vi "ClearLastError.vi"(8 "error in (no error)":errorcluster, 11 "session id in":i32) -> (0 "error out":errorcluster, 3 "session id out":i32)   [LabVIEW 2018, in "libonnx_wrapper.lvlib"]
doc: "/**\n * @brief Очистить сообщение об ошибке для сессии\n * \n * Сбрасывает сохраненное сообщение об ошибке. Полезно после обработки ошибки,\n * чтобы не получить старое сообщение при следующей проверке.\n * \n * @param sessionId [IN] ID сессии\n * \n * @return void\n */\nvoid ClearLastError(int sessionId);"
uses:
  libonnx_wrapper.lvlib
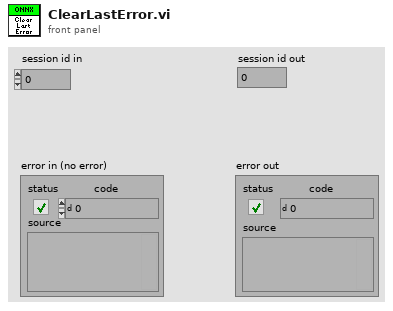
[diagram p1: front panel]
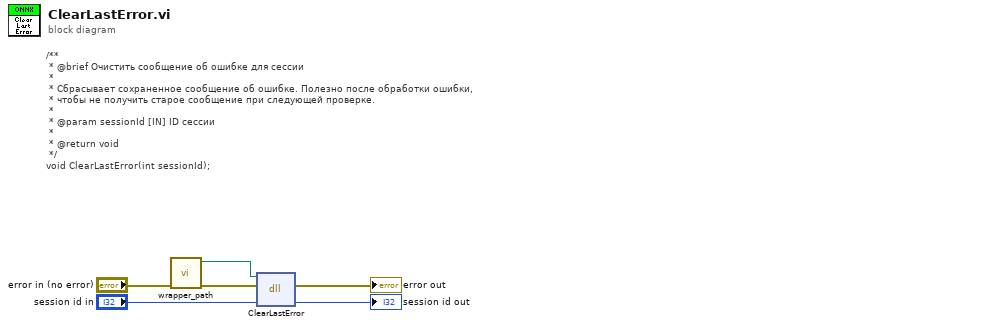
[diagram p0: block diagram]
diagram:
  # "/**\n * @brief Очистить сообщение об ошибке для сессии\n * \n * Сбрасывает сохраненное сообщение об ошибке. Полезно после обработки ошибки,\n * чтобы не получить старое сообщение при следующей проверке.\n * \n * @param sessionId [IN] ID сессии\n * \n * @return void\n */\nvoid ClearLastError(int sessionId);"
  n1 = call "wrapper_path.vi"("error in (no error)"="error in (no error)") -> ("error out"=w4:errorcluster, "wrapper path"=w3:path)  [unwired: 9 in]
  n2 = dll-call lib="home/ivan/LabVIEWData/ONNX/Test/libonnx_wrapper/unix64/libonnx_wrapper.so" fn="ClearLastError"(path in=w3, error in=w4, "sessionId"="session id in") -> (error out=→"error out":errorcluster, "sessionId"=→"session id out":i32)  [unwired: 2 in, 1 out]
